vi "Loop_Image Server.vi"(8 "error in (no error)":errorcluster) -> ()   [LabVIEW 2017, in "VisionSystem.lvlib"]
doc: "This VI is used to send images to the dashboard using the second enet port on the 8 slot controller. This is provided for compatibility, but is higher overhead than using the Camera MJPG approach.\n\nThis software is licensed. Open the labview\\readme\\WPI Robotics Library Open Source License.txt file for more information."
uses:
  VisionSystem.lvlib
  <vilib>/Rock Robotics/WPI/Utilities/Refnum Registry Operation.ctl
  Global_HW Status.vi
  <vilib>/Rock Robotics/Network Tables/NT Write String Array.vi
  <vilib>/Rock Robotics/Network Tables/NT Write String.vi
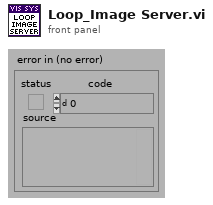
[diagram p1: front panel]
types:
  T1 = enum16{"Standard", "Buffered", "CRLF", "Immediate"}
  T2 = typedef "Refnum Registry Operation.ctl" = enum16{"set", "get", "delete", "get all names", "read name"}
  T3 = cluster{"token string":string, "token string 2":string}[]
  T4 = typedef "VisionSystem.lvlib/Cluster_HW_Status.ctl" = cluster{"Cam Active":bool, "Cam Image":T5, "Cam Setings":T6, "Target":T11, "Camera Ref":T12}
  T5 = typedef "IMAQ Image.ctl" = refnum<image>
  T6 = typedef "Cluster_Camera Settings.ctl" = cluster{"Image Size":T7, "Frame Rate (fps)":T8, "White Balance":T9, "Exposure":T10, "Exposure (%)":dbl, "Brightness":i32, "Sharpness":i32, "Saturation":i32}
  T7 = typedef "WPI_CameraImageSize.ctl" = enum16{"640x480", "320x240", "160x120", "Custom"}
  T8 = typedef "WPI_CameraFrameRate.ctl" = u32
  T9 = typedef "WPI_CameraWhite Balance Values.ctl" = enum16{"Auto", "Fixed indoor", "Fixed outdoor 1", "Fixed outdoor 2", "Fixed fluorescent 1", "Fixed fluorescent 2", "Hold current", "Custom"}
  T10 = typedef "WPI_CameraExposure Values.ctl" = enum16{"Auto", "Flicker-free 50 Hz", "Flicker-free 60 Hz", "Hold current", "Custom"}
  T11 = typedef "VisionSystem.lvlib/Enum_ Field Targets.ctl" = enum16{"Boiler (USB 0)", "Rope (USB 1)"}
  T12 = typedef "WPI_CameraDevRef.ctl" = cluster{"Camera Address":string, "CameraStatus":errorcluster}
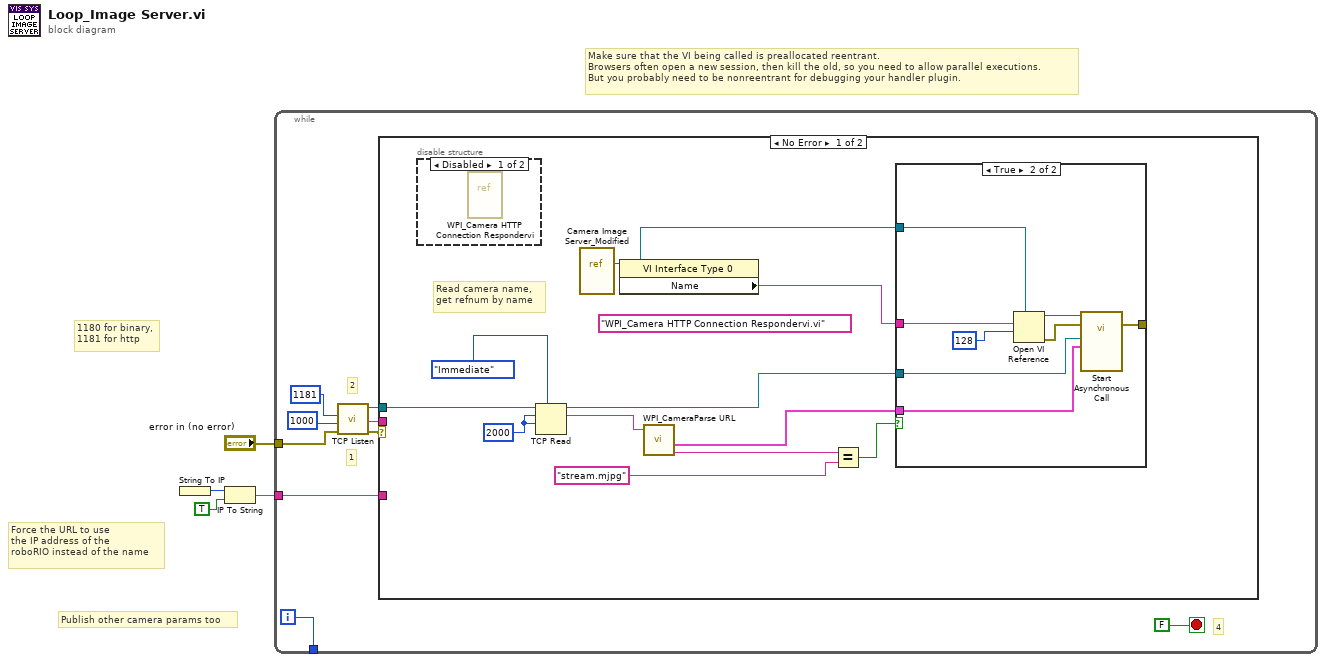
[diagram p0: block diagram]
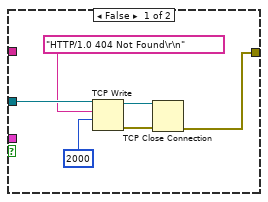
[diagram p3: hidden frame]
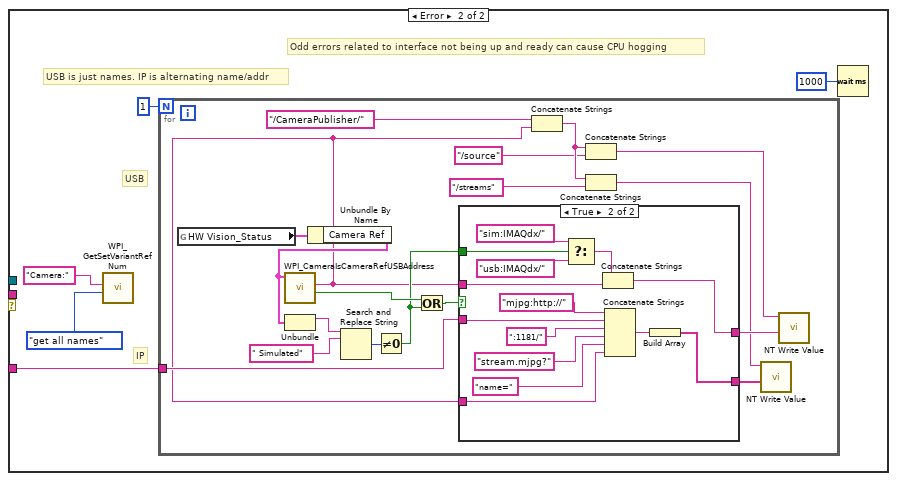
[diagram p4: hidden frame]
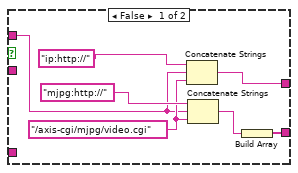
[diagram p5: hidden frame]
diagram:
  # "Force the URL to use\nthe IP address of the\nroboRIO instead of the name"
  # "Make sure that the VI being called is preallocated reentrant.\nBrowsers often open a new session, then kill the old, so you need to allow parallel executions.\nBut you probably need to be nonreentrant for debugging your handler plugin."
  # "Publish other camera params too"
  # "1180 for binary,\n1181 for http"
  n1 = String To IP() -> (0:w2:u32)  [unwired: 1 in]
  n2 = IP To String(1:TRUE ("dot notation? (F)"), 2:w2) -> (0:w3:string)
  n3 = while {
    tunnel: "error in (no error)" -> [w12]
    tunnel: [w7] -> _
    tunnel: w3 -> [w5]
    i -> [w7]
    stop <- FALSE ("status") stop-if-true
    # "4"
    # "1"
    # "2"
    n4 = call <vilib>:"TCP Listen.vi"("error in (no error)"=w12, "timeout ms (wait forever: -1)"=u16 1000 ("port"), "port"=u16 1181) -> ("error out"=w9:errorcluster, "remote address"=w13:string, "connection ID"=w11:refnum<k5>)  [unwired: 1 in, 5 out]
    n5 = case shown="No Error" w9 {
      tunnel: w13 -> [_ _]
      tunnel: w11 -> [w22 _]
      tunnel: w5 -> [_ w40]
      frame No Error {
        w23 = 2000
        (unwired) "WPI_Camera HTTP Connection Respondervi.vi"
        # "Read camera name,\nget refnum by name"
        n6 = disable-structure shown="Disabled" {
          frame Disabled {
            n7 = vi-ref <vilib>:"WPI_Camera HTTP Connection Respondervi.vi"() -> ()  [unwired: 1 out]
          }
          frame Enabled {
          }
        }
        n8 = TCP Read(connection ID=w22, bytes to read=w23, 7:T1."Immediate" ("mode (standard)"), 9:w23) -> (connection ID out=w21:refnum<k5>, data out=w16:string)  [unwired: 1 in, 1 out]
        n9 = vi-ref "Camera Image Server_Modified.vi"() -> (w14:refnum<vi>)
        n10 = property class="VI Interface Type 0"(reference=w14) -> ("Name"=w15:string)  [unwired: 1 in, 2 out]
        n11 = call <vilib>:"WPI_CameraParse URL.vi"("URL"=w16) -> ("cgi string"=w18:string, "parameters"=w17:T3)  [unwired: 7 in, 2 out]
        n12 = Equal?(x=w18, y="stream.mjpg") -> (x = y?=w20:bool)
        n13 = case shown="True" w20 {
          tunnel: w15 -> [_ w38]
          tunnel: w21 -> [w30 w35]
          tunnel: [w25 w33] -> _
          tunnel: w17 -> [_ w32]
          tunnel: w14 -> [_ w31]
          frame False {
            n14 = TCP Write(connection ID=w30, data in="HTTP/1.0 404 Not Found\r\n" ("regular expression"), 9:2000) -> (connection ID out=w29:refnum<k5>, error out=w26:errorcluster)  [unwired: 1 in, 1 out]
            n15 = TCP Close Connection(connection ID=w29, error in (no error)=w26) -> (error out=w25:errorcluster)  [unwired: 2 out]
          }
          frame True {
            n16 = Open VI Reference(type specifier VI Refnum (for type only)=w31, vi path=w38, options=128) -> (vi reference=w36:refnum<vi>, error out=w34:errorcluster)  [unwired: 3 in]
            n17 = call-by-ref "Start Asynchronous Call"(reference=w36, error in=w34, "parameters"=w32, "connection ID"=w35) -> (error out=w33:errorcluster)  [unwired: 10 in, 1 out]
          }
        }
      }
      frame Error {
        # "USB is just names. IP is alternating name/addr"
        # "IP"
        # "USB"
        # "Odd errors related to interface not being up and ready can cause CPU hogging"
        n18 = call <vilib>:"WPI_GetSetVariantRefNum.vi"("Operation"=Refnum_Registry_Operation."get all names" ("menu"), "refnum name"="Camera:") -> ()  [unwired: 7 in, 3 out]
        n19 = for {
          N: 1 -> [_]
          tunnel: w40 -> [w61]
          n20 = global read "Global_HW Status.vi" "HW Vision_Status"() -> (w46:T4)
          n21 = Unbundle By Name(w46) -> ("Camera Ref"=w45:T12)
          n22 = call <vilib>:"WPI_CameraIsCameraRefUSBAddress.vi"("CameraDevRef"=w45) -> ("USB?"=w49:bool, "Camera Address Out"=w44:string)  [unwired: 7 in, 2 out]
          n23 = Unbundle(w45) -> ("Camera Address"=w51:string)  [unwired: 1 out]
          n24 = Search and Replace String(input string=w51, search string=" Simulated") -> (number of replacements=w50:i32)  [unwired: 6 in, 3 out]
          n25 = Not Equal To 0?(x=w50) -> (x != 0?=w47:bool)
          n26 = Or(x=w49, y=w47) -> (x .or. y?=w48:bool)
          n27 = case shown="True" w48 {
            tunnel: w44 -> [w64 w74]
            tunnel: w61 -> [_ w81]
            tunnel: w44 -> [_ w77]
            tunnel: [w62 w73] -> w60
            tunnel: [w66 w75] -> w53
            tunnel: w47 -> [_ w72]
            frame False {
              w65 = "/axis-cgi/mjpg/video.cgi"
              n28 = Concatenate Strings("ip:http://", w64, w65) -> (w62:string)
              n29 = Concatenate Strings("mjpg:http://", w64, w65) -> (w67:string)
              n30 = Build Array(w67) -> (w66:string[])
            }
            frame True {
              n31 = Select(t="sim:IMAQdx/", s=w72, f="usb:IMAQdx/") -> (s? t:f=w69:string)
              n32 = Concatenate Strings(w69, w74) -> (w73:string)
              n33 = Concatenate Strings("mjpg:http://", w81, ":1181/", "stream.mjpg?", "name=", w77) -> (w76:string)
              n34 = Build Array(w76) -> (w75:string[])
            }
          }
          n35 = Concatenate Strings("/CameraPublisher/", w44) -> (w57:string)
          n36 = Concatenate Strings(w57, "/source") -> (w54:string)
          n37 = Concatenate Strings(w57, "/streams") -> (w55:string)
          n38 = call-poly <vilib>:"NT Write Value.vi"("String Array"=w53, "Name"=w55) -> ()  [unwired: 9 in, 1 out]
          n39 = call-poly <vilib>:"NT Write Value.vi"("String"=w60, "Name"=w54) -> ()  [unwired: 9 in, 1 out]
        }
        n40 = Wait (ms)(milliseconds to wait=u32 1000) -> ()  [unwired: 1 out]
      }
    }
  }
